vi "Initialize TDK 20-38.vi"(8 "error in (no error)":errorcluster, 11 "NI MAX name":string) -> (0 "error out":errorcluster, 3 "VISA out":refnum<visa-resource-name>)   [LabVIEW 2023, in "TDK20-38 API.lvlib"]
uses:
  TDK20-38 API.lvlib
  LabVIEW - Drivers/Genesys Drivers/LAN/TDK-Lambda GEN LAN Series.lvlib
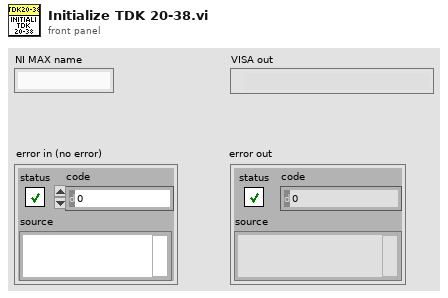
[diagram p1: front panel]
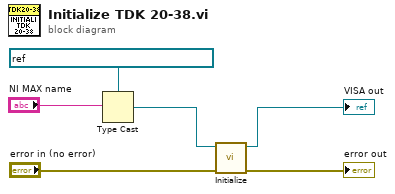
[diagram p0: block diagram]
diagram:
  n1 = Type Cast(type=refnum<visa-resource-name> "TCPIP0::192.168.0.17::inst0::INSTR" ("VISA name"), x="NI MAX name") -> (*(type *) &x=w1:refnum<visa-resource-name>)
  n2 = call "Initialize.vi"("error in (no error)"="error in (no error)", "VISA name"=w1) -> ("error out"=→"error out":errorcluster, "VISA out"=→"VISA out":refnum<visa-resource-name>)  [unwired: 8 in]
